vi "GenerateAttachablePosition_Rook.vi"(1 "Castling State":bool[][](array[boolean]), 2 "Black/White Turn (T/F)":bool, 3 "Board":i32[][](array[numeric])=[[-3, 0, 0, 0, -1, -4, -5, -3], [0, -6, -6, -6, -6, -6, -6, 0], [0, 0, 0, 0, 0, 0, 0, 0], [0, 0, 0, 0, 0, 0, 0, 0], [0, 0, 0, 0, 0, 0, 0, 0], [0, 0, 0, 0, 0, 0, 0, 0], [0, 6, 6, 6, 6, 6, 6, 0], [3, 0, 0, 0, 1, 0, 0, 3]], 4 "pieceIndex":i32) -> (0 "AttachablePosition":bool[][](array[boolean]))   [LabVIEW 2014]
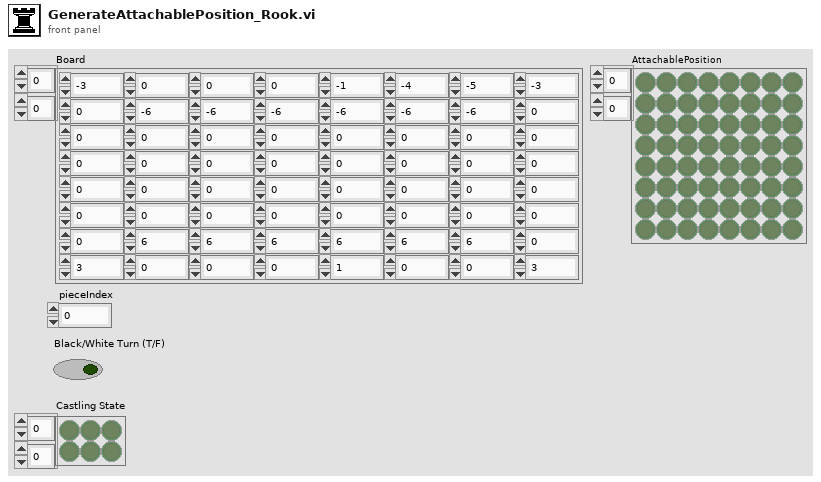
[diagram p1: front panel]
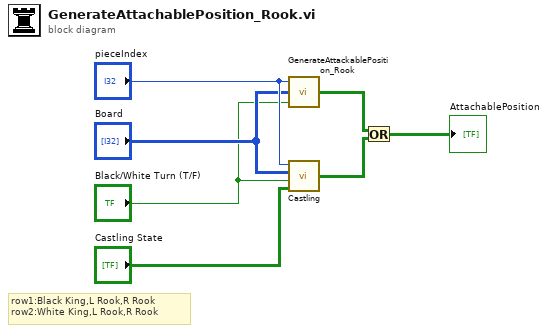
[diagram p0: block diagram]
diagram:
  # "row1:Black King,L Rook,R Rook\nrow2:White King,L Rook,R Rook"
  n1 = call "GenerateAttackablePosition_Rook.vi"("Black/White Turn (T/F)"="Black/White Turn (T/F)", "Board"="Board", "pieceIndex"="pieceIndex") -> ("AttachablePosition"=w2:bool[][])
  n2 = call "Castling.vi"("Castling State"="Castling State", "Black/White Turn (T/F)"="Black/White Turn (T/F)", "Board"="Board", "pieceIndex"="pieceIndex") -> ("Castling position"=w3:bool[][])
  n3 = Or(x=w2, y=w3) -> (x .or. y?=→"AttachablePosition":bool[][])
